vi "IPS - USE - 1.vi"() -> ()   [LabVIEW 2013, in "Mercury iXX.lvlib"]
uses:
  <instrlib>/Mercury iXX/Mercury iXX.lvlib
  <instrlib>/Mercury iXX/Public/Controls/ISOBus Address.ctl
  <instrlib>/Mercury iXX/Public/Controls/Serial Settings.ctl
  <instrlib>/Mercury iXX/Public/Controls/Comms Transport Layer.ctl
  <instrlib>/Mercury iXX/Public/Libraries/Magnet/Controls/PSU Actions.ctl
  <instrlib>/Mercury iXX/Public/Libraries/Magnet.lvlib
panel:
  in  "HOLD":bool
  out "SW HTR\nCONFIRM":bool
  in  "SWITCH\nHEATER":bool
  out "PSU Act Stat 2":T1 caption="Mode Status"
  out "Output Voltage (V)":dbl format="%.4g"
  out "Output Current (A)":dbl format="%.4g"
  in  "stop":bool
  in  "IP Address":string
  in  "Target Rate (T/min)":dbl
  in  "Target Field (T)":dbl
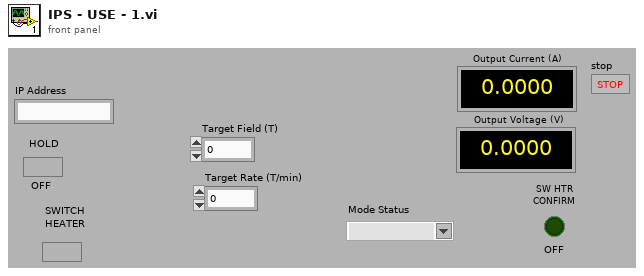
[diagram p1: front panel]
types:
  T1 = typedef "Mercury iXX.lvlib/Magnet.lvlib/PSU Actions.ctl" = string
  T2 = typedef "Mercury iXX.lvlib/Comms Transport Layer.ctl" = enum16{"Ethernet TCP/IP", "USB", "ISOBus - RS-232", "GPIB"}
  T3 = typedef "Mercury iXX.lvlib/Serial Settings.ctl" = cluster{"Baud Rate":u32, "Parity":u16, "Data Bits":u16, "Stop Bits":u16, "Flow Control":u16}
  T4 = typedef "Mercury iXX.lvlib/ISOBus Address.ctl" = i32
  T5 = cluster{"VISA resource name":refnum<visa-resource-name>, "Comms Layer":T2, "IP Address":string, "Serial Configuration":T3, "ISOBUS address":T4}
  T6 = cluster{"Target Current (A)":dbl, "Target Rate (A/min)":dbl, "SEND TO IPS":bool, "Target Field (T)":dbl, "Target Rate (T/min)":dbl}
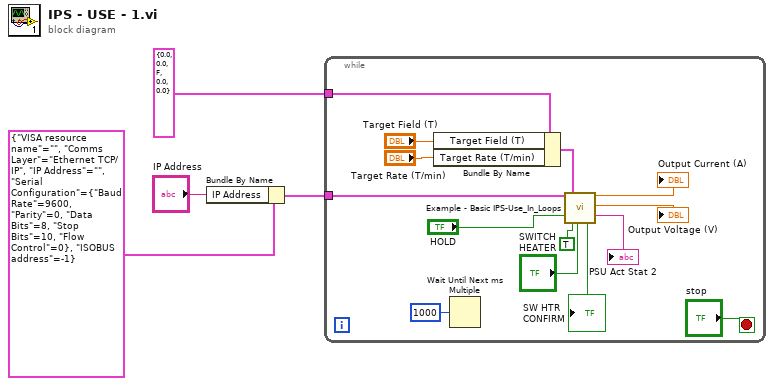
[diagram p0: block diagram]
diagram:
  n1 = Bundle By Name(cluster=T5 {"VISA resource name"="", "Comms Layer"=enum."Ethernet TCP/IP", "IP Address"="", "Serial Configuration"={"Baud Rate"=9600, "Parity"=0, "Data Bits"=8, "Stop Bits"=10, "Flow Control"=0}, "ISOBUS address"=-1} ("Connection Details"), "IP Address"="IP Address") -> (w1:T5)
  n2 = while {
    tunnel: T6 {"Target Current (A)"=0.0, "Target Rate (A/min)"=0.0, "SEND TO IPS"=FALSE, "Target Field (T)"=0.0, "Target Rate (T/min)"=0.0} ("Ramp Controls") -> [w18]
    tunnel: w1 -> [w13]
    stop <- "stop" stop-if-true
    n3 = Bundle By Name(cluster=w18, "Target Field (T)"="Target Field (T)", "Target Rate (T/min)"="Target Rate (T/min)") -> (w17:T6)
    n4 = Wait Until Next ms Multiple(millisecond multiple=u32 1000) -> ()  [unwired: 1 out]
    n5 = call <instrlib>:"Example - Basic IPS-Use_In_Loops.vi"("Connection Details"=w13, "HOLD"="HOLD", "Ramp Controls"=w17, "AMP/TESLA"=TRUE, "SWITCH\nHEATER"="SWITCH\nHEATER") -> ("SW HTR\nCONFIRM"=→"SW HTR\nCONFIRM":bool, "Output Current (A)"=→"Output Current (A)":dbl, "Output Voltage (V)"=→"Output Voltage (V)":dbl, "PSU Act Stat 2"=→"PSU Act Stat 2":T1)  [unwired: 5 in, 6 out]
  }
